vi "PacketParse7.vi"(0 "Packet array in":u8[](array[numeric])) -> (1 "Data Point":cluster{"time":u32, "value":sgl}, 2 "Data ID":u32)   [LabVIEW 2015]
panel:
  # "PacketParser takes in an array of  10 bytes and converts it into a data point bundle\ncomprised of a 32-bit unsigned integer time stamp and a single-precision float, along with\na data ID."
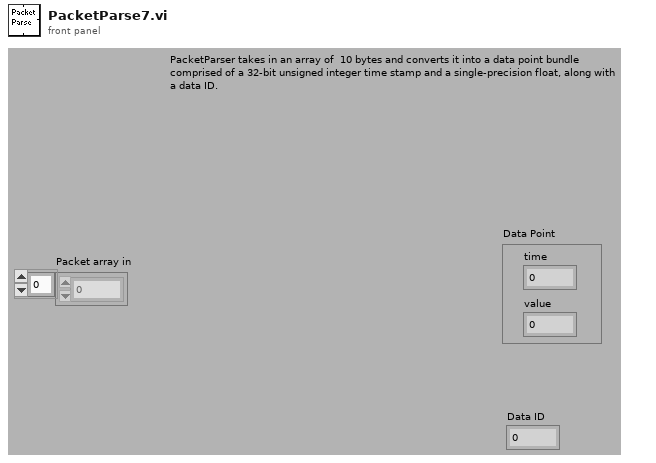
[diagram p1: front panel]
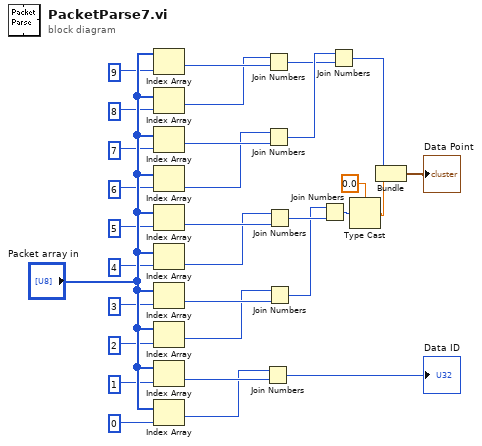
[diagram p0: block diagram]
diagram:
  n1 = Index Array(array="Packet array in", index=9) -> (element=w25:u8)
  n2 = Index Array(array="Packet array in", index=8) -> (element=w24:u8)
  n3 = Index Array(array="Packet array in", index=7) -> (element=w23:u8)
  n4 = Index Array(array="Packet array in", index=6) -> (element=w22:u8)
  n5 = Index Array(array="Packet array in", index=5) -> (element=w21:u8)
  n6 = Index Array(array="Packet array in", index=4) -> (element=w20:u8)
  n7 = Index Array(array="Packet array in", index=3) -> (element=w19:u8)
  n8 = Index Array(array="Packet array in", index=2) -> (element=w18:u8)
  n9 = Index Array(array="Packet array in", index=1) -> (element=w17:u8)
  n10 = Index Array(array="Packet array in", index=0) -> (element=w16:u8)
  n11 = Join Numbers(hi=w16, lo=w17) -> ((hi.lo)=→"Data ID":u16)
  n12 = Join Numbers(hi=w24, lo=w25) -> ((hi.lo)=w28:u16)
  n13 = Join Numbers(hi=w22, lo=w23) -> ((hi.lo)=w29:u16)
  n14 = Join Numbers(hi=w20, lo=w21) -> ((hi.lo)=w31:u16)
  n15 = Join Numbers(hi=w18, lo=w19) -> ((hi.lo)=w30:u16)
  n16 = Join Numbers(hi=w30, lo=w31) -> ((hi.lo)=w27:u32)
  n17 = Join Numbers(hi=w29, lo=w28) -> ((hi.lo)=w14:u32)
  n18 = Type Cast(type=sgl 0.0, x=w27) -> (*(type *) &x=w15:sgl)
  n19 = Bundle(w14, w15) -> (→"Data Point":cluster{u32, sgl})  [unwired: 1 in]
